vi "main.vi"() -> ()   [LabVIEW 2014]
uses:
  <vilib>/Instr/_visa.llb/VISA Configure Serial Port (Instr).vi
  <instrlib>/Keithley 24XX/Public/Data/Read (Single Point).vi
  <instrlib>/Keithley 24XX/Keithley 24XX.lvlib
panel:
  out "Seconds":sgl
  out "Chamber *C Data":string
  in  "Chamber *C Data":path=path "C:/Users/Administrator/Documents/humidity_sensing_setup/data/dumb/chamber_c_data.txt"
  out "Chamber *C Graph":sgl(graph)=5460.51
  out "Chamber *C":sgl
  out "Thermocouple Temperature Graph":sgl(graph)=5460.51
  out "Thermocouple Temperature":sgl
  out "Thermocouple *C Data":string
  in  "Thermocouple *C Data":path=path "C:/Users/Administrator/Documents/humidity_sensing_setup/data/dumb/thermocouple_c_data.txt"
  out "Pressure Data":string
  in  "Pressure Data":path=path "C:/Users/Administrator/Documents/humidity_sensing_setup/data/dumb/pressure_data.txt"
  out "Pressure Graph":sgl(graph)=5460.51
  out "Pressure":sgl
  in  "Start Button":bool
  in  "Operation Mode":bool
  out "Humidity":sgl
  out "Humidity Data":string
  in  "Humidity Data":path=path "C:/Users/Administrator/Documents/humidity_sensing_setup/data/dumb/humidity_data.txt"
  out "Humidity Data Graph":sgl(graph)=5460.51
  out "Resistance Data":string
  in  "Resistance Data":path=path "C:/Users/Administrator/Documents/humidity_sensing_setup/data/dumb/resistance_data.txt"
  out "Current Data":string
  in  "Current Data":path=path "C:/Users/Administrator/Documents/humidity_sensing_setup/data/dumb/current_data.txt"
  in  "Sampling rate (ms/pt)":i32=1000
  in  "Stop Voltage/Current":dbl=1.0
  in  "Start Voltage/Current":dbl=1.0
  in  "current multiplier":dbl=1000000.0
  in  "stop button":bool
  out "Current Data Graph":sgl(graph)=0.0001831192
  out "Resistance Data Graph":sgl(graph)=5460.51
  in  "loop num":dbl=10000000000.0
  in  "Step":dbl
  in  "Source Mode  (0: Voltage)":u16(ring) items=["Voltage", "Current"]
  in  "Compliance  Level (0.1)":dbl=1.0
  in  "Enable Resistance Auto R. (T:Enable)":bool
  in  "Enable Current Auto R. (T:Enable)":bool=TRUE
  in  "Enable Voltage Auto R. (T:Enable)":bool
  in  "Resistance M. R. (1.0)":dbl=1.0
  in  "Current M. Range (1.0)":dbl=1.0
  in  "Voltage M. Range (1.0)":dbl=1.0
  out "Resistance":sgl
  out "Current":sgl
  out "Voltage":sgl
  in  "Serial Configuration":T1={"Baud Rate"=9600, "Parity"=0, "Data Bits"=8, "Stop Bits"=10, "Flow Control"=0} {"Flow Control" items=["None", "XON/XOFF", "RTS/CTS", "XON/XOFF & RTS/CTS", "DTR/DSR", "XON/XOFF & DTR/DSR"]; "Stop Bits" items=["1.0"=10, "1.5"=15, "2.0"=20]; "Data Bits" items=["7"=7, "8"=8]; "Parity" items=["None", "Odd", "Even", "Mark", "Space"]; "Baud Rate" items=["300"=300, "600"=600, "1200"=1200, "2400"=2400, "4800"=4800, "9600"=9600, "19200"=19200]}
  in  "Keithley VISA resource name":refnum<visa-resource-name>="GPIB9::24::INSTR"
  out "Arduino Status":bool
  out "error out":errorcluster
  in  "error in":errorcluster
  in  "instr name":string="Arduino"
  in  "write":bool
  in  "buffer size":u32=256
  in  "timeout (ms)":u32=10000
  in  "flow control":u16
  in  "stop bits":u16=10
  in  "parity":u16(ring) items=["None", "Odd", "Even", "Mark", "Space"]
  in  "data bits":u16=8 min=5 max=8 step=1
  in  "baud rate":u32=9600
  in  "write string":string
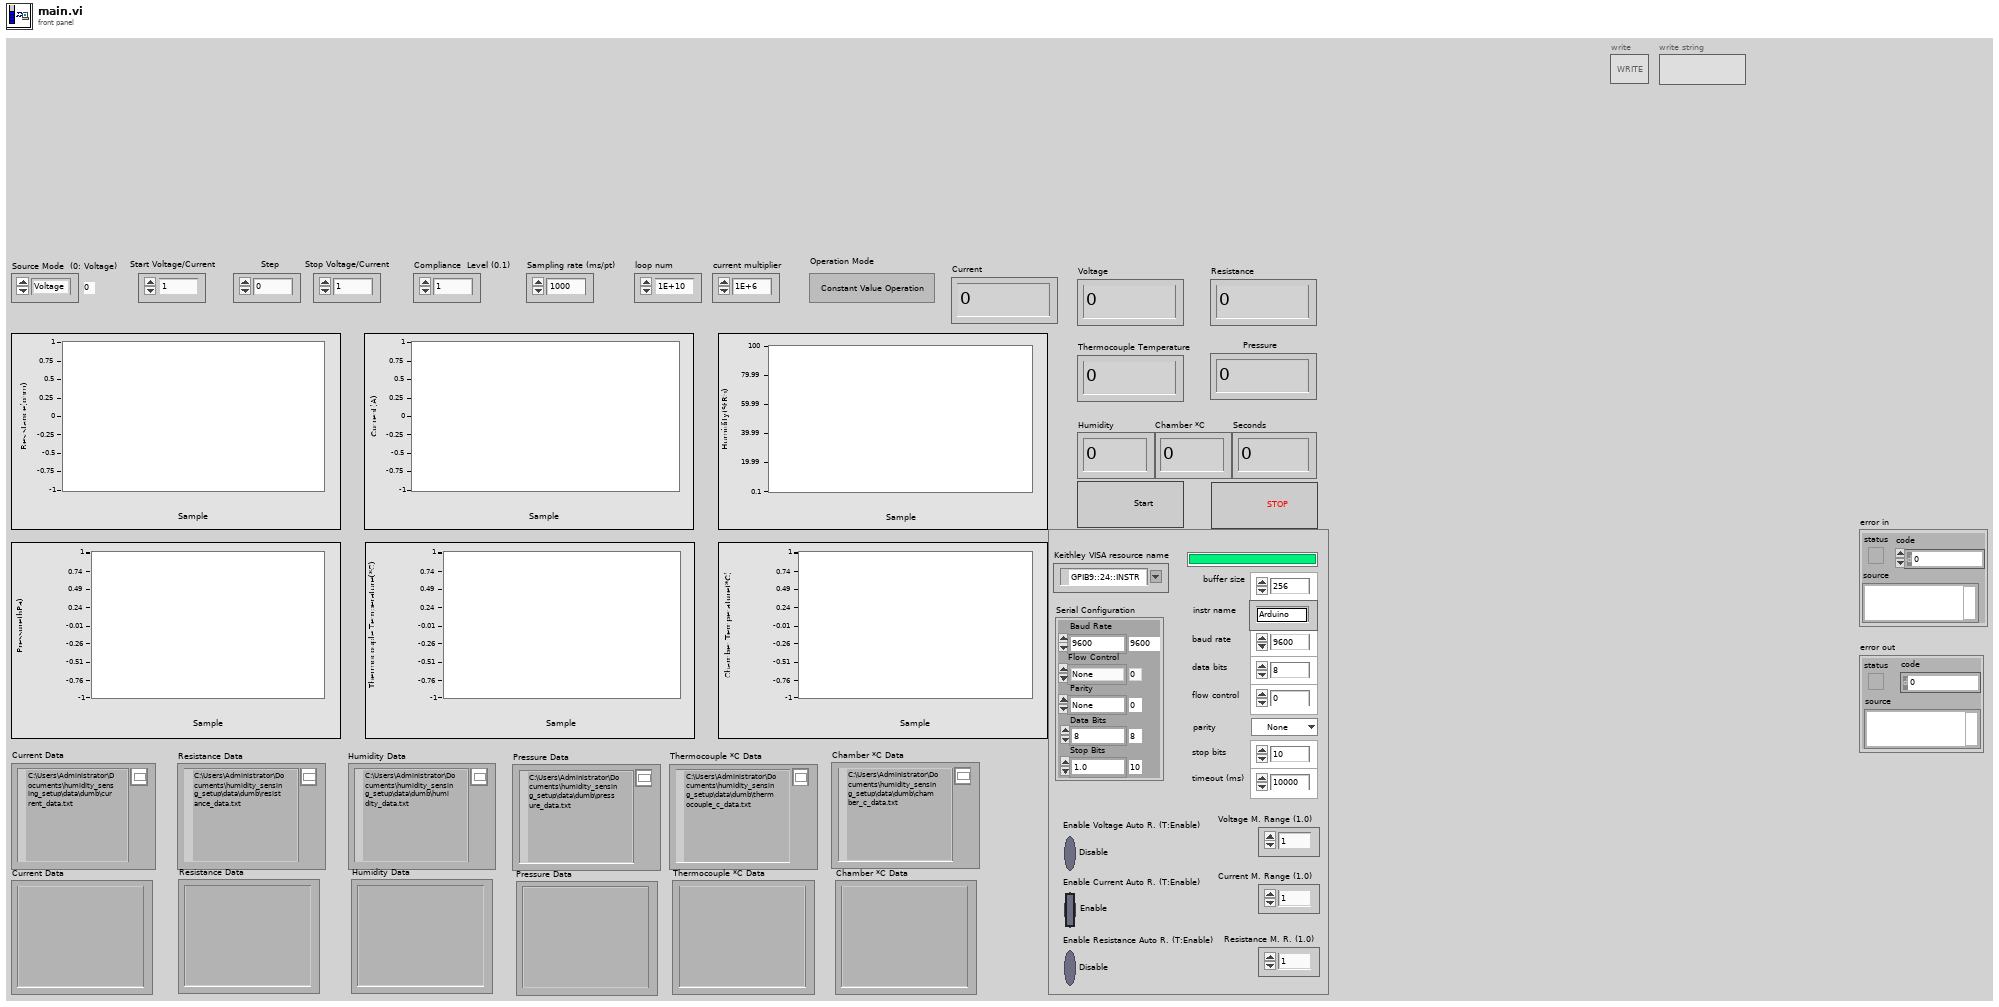
[diagram p1: front panel]
types:
  T1 = cluster{"Baud Rate":u32, "Parity":u16, "Data Bits":u16, "Stop Bits":u16, "Flow Control":u16}
  T2 = enum16{"open", "replace", "create", "open or create", "replace or create", "replace or create with confirmation"}
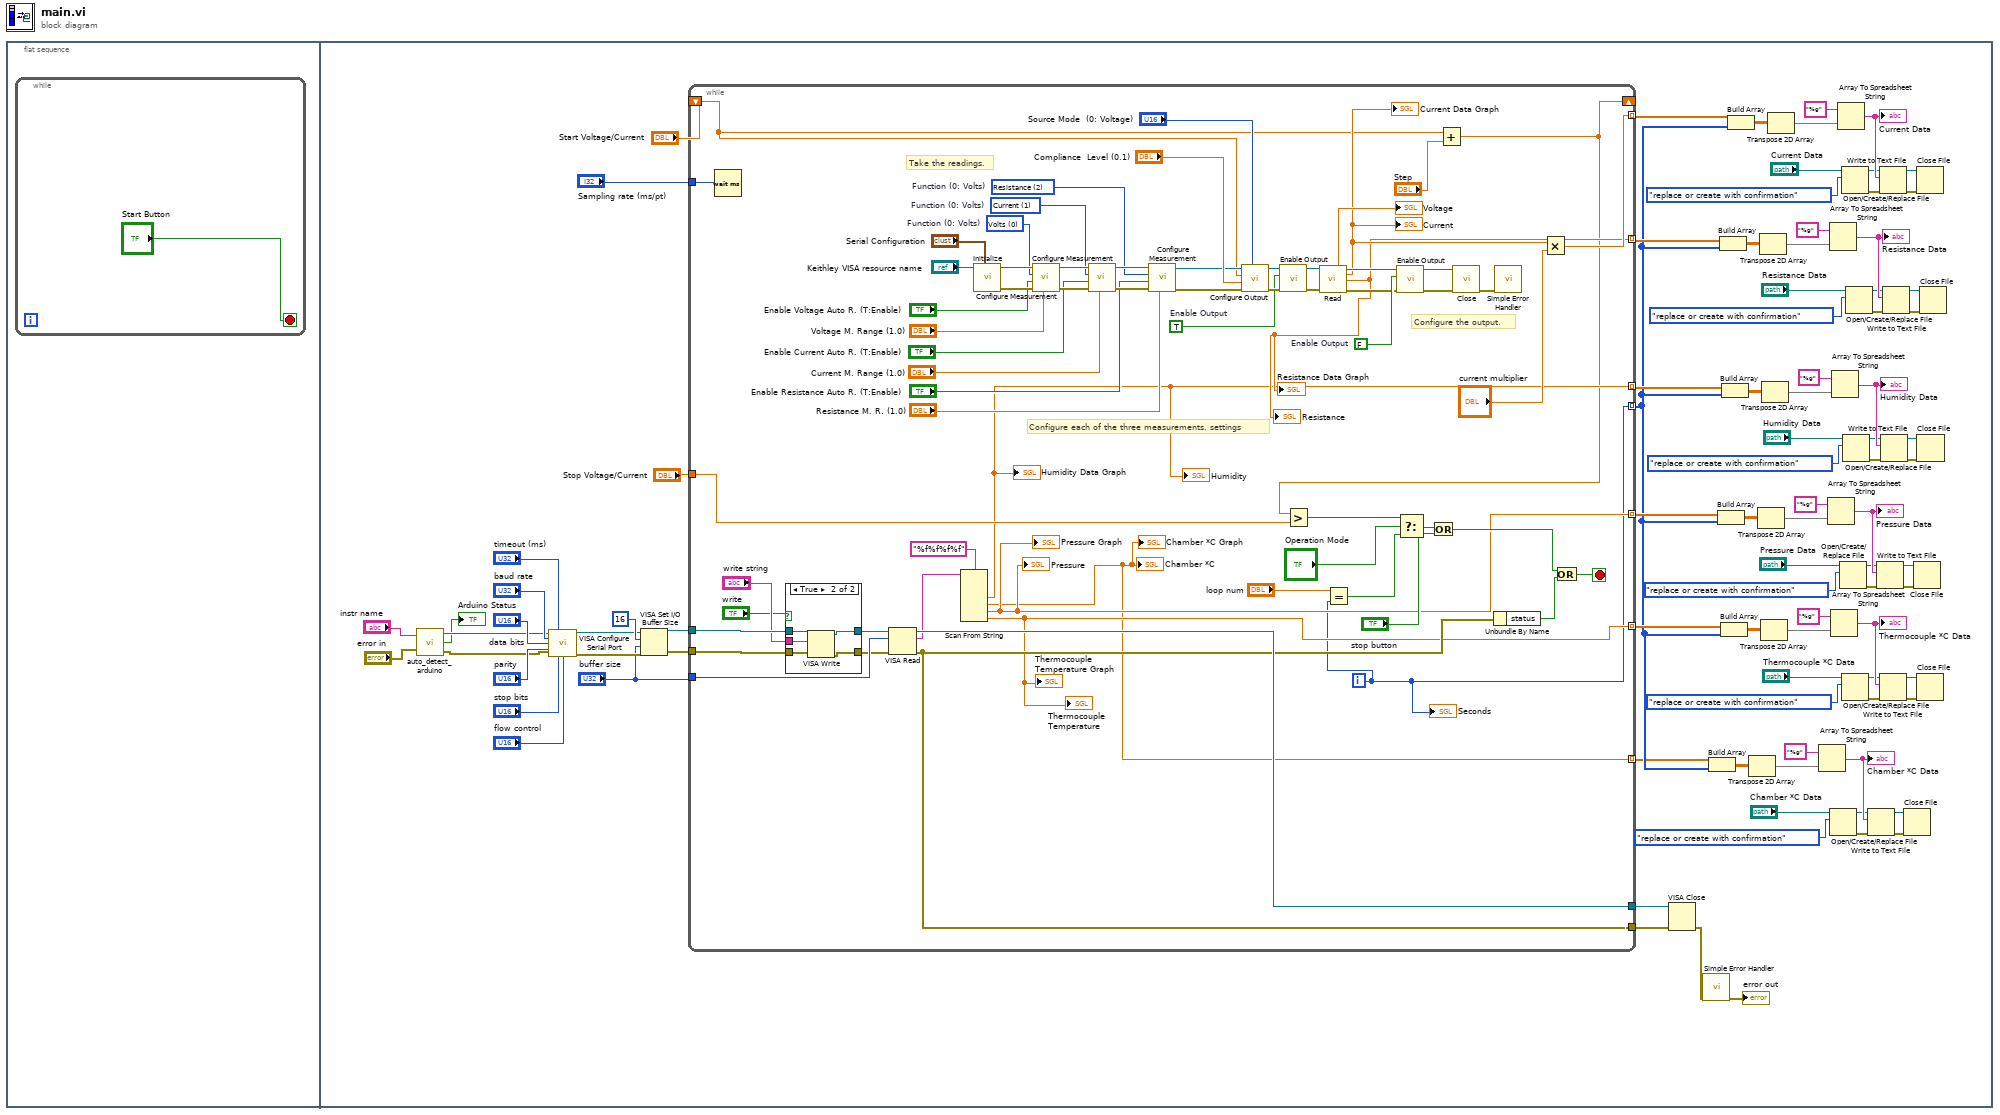
[diagram p0: block diagram]
diagram:
  n1 = flat-sequence {
    frame #0 {
      n2 = while {
        stop <- "Start Button" stop-if-true
      }
    }
    frame #1 {
      n3 = call "auto_detect_arduino.vi"("instr name"="instr name", "error in"="error in") -> ("VISA resource name"=w84:refnum<visa-resource-name>, "status"=→"Arduino Status":bool, "error out"=w83:errorcluster)
      n4 = call-poly "VISA Configure Serial Port"("VISA resource name"=w84, "timeout (10sec)"="timeout (ms)", "baud rate (9600)"="baud rate", "data bits (8)"="data bits", "parity (0:none)"="parity", "error in (no error)"=w83, "stop bits (10: 1 bit)"="stop bits", "flow control (0:none)"="flow control") -> ("VISA resource name out"=w80:refnum<visa-resource-name>, "error out"=w79:errorcluster)  [unwired: 6 in]
      n5 = VISA Set I/O Buffer Size(VISA resource name=w80, mask (16)=u16 16 ("I/O Receive\nBuffer mask"), size (4096)="buffer size", error in (no error)=w79) -> (VISA resource name out=w78:refnum<visa-resource-name>, error out=w77:errorcluster)
      n6 = while {
        tunnel: w78 -> [w156]
        tunnel: w77 -> [w155]
        tunnel: [w157] -> w92
        tunnel: [w100] -> w91
        tunnel: "buffer size" -> [w158]
        tunnel: [w102] -> w36 mode=indexing
        tunnel: "Sampling rate (ms/pt)" -> [w112]
        tunnel: "Stop Voltage/Current" -> [w111]
        tunnel: [w110] -> w49 mode=indexing
        tunnel: [w93] -> w3 mode=indexing
        tunnel: [w109] -> w48 mode=indexing
        shift-right: [w101] -> _
        shift-left: "Start Voltage/Current" -> [w108]
        tunnel: [w96] -> w25 mode=indexing
        tunnel: [w95] -> w14 mode=indexing
        tunnel: [w94] -> w2 mode=indexing
        i -> [w93]
        stop <- w159 stop-if-true
        w121 = TRUE  # Enable Output
        w131 = FALSE  # Enable Output
        w138 = u16 2 items=["Volts", "Current", "Resistance"]  # Function (0: Volts)
        w139 = u16 1 items=["Volts", "Current", "Resistance"]  # Function (0: Volts)
        w140 = u16 0 items=["Volts", "Current", "Resistance"]  # Function (0: Volts)
        # "Take the readings."
        # "Configure the output."
        # "Configure each of the three measurements. settings"
        n7 = Wait (ms)(milliseconds to wait=w112) -> ()  [unwired: 1 out]
        n8 = case shown="True" "write" {
          tunnel: w156 -> [w161 w166]
          tunnel: w155 -> [w160 w165]
          tunnel: [w161 w164] -> w154
          tunnel: [w160 w163] -> w153
          tunnel: "write string" -> [_ w162]
          frame False {
          }
          frame True {
            n9 = VISA Write(VISA resource name=w166, write buffer=w162, error in (no error)=w165) -> (VISA resource name out=w164:refnum<visa-resource-name>, error out=w163:errorcluster)  [unwired: 1 out]
          }
        }
        n10 = VISA Read(VISA resource name=w154, byte count=w158, error in (no error)=w153) -> (VISA resource name out=w157:refnum<visa-resource-name>, read buffer=w97:string, error out=w100:errorcluster)  [unwired: 1 out]
        n11 = Scan From String(format string="%f%f%f%f", input string=w97) -> (output 1=w102:sgl, output 2=w94:sgl, output 3=w96:sgl, output 4=w95:sgl)  [unwired: 6 in, 3 out]
        "Humidity Data Graph" <- w102
        "Humidity" <- w102
        "Pressure" <- w96
        "Pressure Graph" <- w96
        "Thermocouple Temperature" <- w95
        "Thermocouple Temperature Graph" <- w95
        "Chamber *C" <- w94
        "Chamber *C Graph" <- w94
        n12 = call <instrlib>:"Initialize.vi"("Serial Configuration"="Serial Configuration", "VISA resource name"="Keithley VISA resource name") -> ("error out"=w145:errorcluster, "VISA resource name out"=w146:refnum<visa-resource-name>)  [unwired: 8 in]
        n13 = call <instrlib>:"Configure Measurement.vi"("Manual Range (1.0)"="Voltage M. Range (1.0)", "error in (no error)"=w145, "Enable Auto Range (T:Enable)"="Enable Voltage Auto R. (T:Enable)", "Function (0: Volts)"=w140, "VISA resource name"=w146) -> ("error out"=w143:errorcluster, "VISA resource name out"=w144:refnum<visa-resource-name>)  [unwired: 5 in]
        n14 = call <instrlib>:"Configure Measurement.vi"("Manual Range (1.0)"="Current M. Range (1.0)", "error in (no error)"=w143, "Enable Auto Range (T:Enable)"="Enable Current Auto R. (T:Enable)", "Function (0: Volts)"=w139, "VISA resource name"=w144) -> ("error out"=w142:errorcluster, "VISA resource name out"=w141:refnum<visa-resource-name>)  [unwired: 5 in]
        n15 = call <instrlib>:"Configure Measurement.vi"("Manual Range (1.0)"="Resistance M. R. (1.0)", "error in (no error)"=w142, "Enable Auto Range (T:Enable)"="Enable Resistance Auto R. (T:Enable)", "Function (0: Volts)"=w138, "VISA resource name"=w141) -> ("error out"=w120:errorcluster, "VISA resource name out"=w119:refnum<visa-resource-name>)  [unwired: 5 in]
        n16 = call <instrlib>:"Configure Output.vi"("Source Mode  (0: Voltage)"="Source Mode  (0: Voltage)", "error in (no error)"=w120, "Compliance  Level (0.1)"="Compliance  Level (0.1)", "Output Level (0)"=w108, "VISA resource name"=w119) -> ("error out"=w122:errorcluster, "VISA resource name out"=w123:refnum<visa-resource-name>)  [unwired: 5 in]
        n17 = call <instrlib>:"Enable Output.vi"("error in (no error)"=w122, "Enable Output (T: Enable)"=w121, "VISA resource name"=w123) -> ("error out"=w125:errorcluster, "VISA resource name out"=w124:refnum<visa-resource-name>)  [unwired: 7 in]
        n18 = call-poly <instrlib>:"Read.vi"("VISA resource name"=w124, "error in (no error)"=w125) -> ("Voltage"=→"Voltage":sgl, "VISA resource name out"=w126:refnum<visa-resource-name>, "Current"=w114:sgl, "Resistance"=w109:sgl, "error out"=w127:errorcluster)  [unwired: 7 in, 2 out]
        "Current" <- w114
        "Resistance" <- w109
        "Resistance Data Graph" <- w109
        "Current Data Graph" <- w114
        n19 = Equal?(x="loop num", y=w93) -> (x = y?=w103:bool)
        n20 = call <instrlib>:"Enable Output.vi"("error in (no error)"=w127, "Enable Output (T: Enable)"=w131, "VISA resource name"=w126) -> ("error out"=w128:errorcluster, "VISA resource name out"=w129:refnum<visa-resource-name>)  [unwired: 7 in]
        n21 = Add(x=w108, y="Step") -> (x+y=w101:dbl)
        n22 = Greater?(x=w101, y=w111) -> (0:w106:bool)
        n23 = Select(t=w106, s="Operation Mode", f=w103) -> (s? t:f=w105:bool)
        n24 = Or(x=w105, y="stop button") -> (x .or. y?=w98:bool)
        n25 = call <instrlib>:"Close.vi"("error in (no error)"=w128, "VISA resource name"=w129) -> ("error out"=w149:errorcluster)  [unwired: 9 in]
        n26 = Unbundle By Name(w100) -> ("status"=w99:bool)
        n27 = call <vilib>:"Simple Error Handler.vi"("error in (no error)"=w149) -> ()  [unwired: 4 in, 5 out]
        n28 = Multiply(x=w114, y="current multiplier") -> (x*y=w110:dbl)
        n29 = Or(x=w98, y=w99) -> (x .or. y?=w159:bool)
        "Seconds" <- w93
      }
      n30 = VISA Close(VISA resource name=w92, error in (no error)=w91) -> (error out=w74:errorcluster)
      n31 = call <vilib>:"Simple Error Handler.vi"("error in (no error)"=w74) -> ("error out"=→"error out":errorcluster)  [unwired: 4 in, 4 out]
      n32 = Build Array(w2, w3) -> (w4:sgl[][])
      n33 = Build Array(w25, w3) -> (w26:sgl[][])
      n34 = Build Array(w48, w3) -> (w50:sgl[][])
      n35 = Build Array(w14, w3) -> (w15:sgl[][])
      n36 = Build Array(w36, w3) -> (w37:sgl[][])
      n37 = Build Array(w49, w3) -> (w66:dbl[][])
      n38 = Transpose 2D Array(2D array=w4) -> (transposed array=w12:sgl[][])
      n39 = Transpose 2D Array(2D array=w26) -> (transposed array=w34:sgl[][])
      n40 = Transpose 2D Array(2D array=w50) -> (transposed array=w58:sgl[][])
      n41 = Transpose 2D Array(2D array=w15) -> (transposed array=w23:sgl[][])
      n42 = Transpose 2D Array(2D array=w37) -> (transposed array=w45:sgl[][])
      n43 = Transpose 2D Array(2D array=w66) -> (transposed array=w68:dbl[][])
      n44 = Array To Spreadsheet String(array=w12, 3:"%g" ("format string")) -> (spreadsheet string=w13:string)  [unwired: 1 in]
      "Chamber *C Data" <- w13
      n45 = Array To Spreadsheet String(array=w34, 3:"%g" ("format string")) -> (spreadsheet string=w35:string)  [unwired: 1 in]
      "Pressure Data" <- w35
      n46 = Array To Spreadsheet String(array=w58, 3:"%g" ("format string")) -> (spreadsheet string=w59:string)  [unwired: 1 in]
      "Resistance Data" <- w59
      n47 = Open/Create/Replace File(file path (use dialog)="Chamber *C Data", operation (0:open)=T2."replace or create with confirmation") -> (refnum out=w10:refnum<file>, error out=w5:errorcluster)  [unwired: 4 in, 1 out]
      n48 = Array To Spreadsheet String(array=w23, 3:"%g" ("format string")) -> (spreadsheet string=w24:string)  [unwired: 1 in]
      "Thermocouple *C Data" <- w24
      n49 = Array To Spreadsheet String(array=w45, 3:"%g" ("format string")) -> (spreadsheet string=w46:string)  [unwired: 1 in]
      "Humidity Data" <- w46
      n50 = Array To Spreadsheet String(array=w68, 3:"%g" ("format string")) -> (spreadsheet string=w69:string)  [unwired: 1 in]
      "Current Data" <- w69
      n51 = Open/Create/Replace File(file path (use dialog)="Pressure Data", operation (0:open)=T2."replace or create with confirmation") -> (refnum out=w32:refnum<file>, error out=w27:errorcluster)  [unwired: 4 in, 1 out]
      n52 = Open/Create/Replace File(file path (use dialog)="Current Data", operation (0:open)=T2."replace or create with confirmation") -> (refnum out=w65:refnum<file>, error out=w60:errorcluster)  [unwired: 4 in, 1 out]
      n53 = Open/Create/Replace File(file path (use dialog)="Thermocouple *C Data", operation (0:open)=T2."replace or create with confirmation") -> (refnum out=w21:refnum<file>, error out=w16:errorcluster)  [unwired: 4 in, 1 out]
      n54 = Open/Create/Replace File(file path (use dialog)="Humidity Data", operation (0:open)=T2."replace or create with confirmation") -> (refnum out=w43:refnum<file>, error out=w38:errorcluster)  [unwired: 4 in, 1 out]
      n55 = Open/Create/Replace File(file path (use dialog)="Resistance Data", operation (0:open)=T2."replace or create with confirmation") -> (refnum out=w56:refnum<file>, error out=w51:errorcluster)  [unwired: 4 in, 1 out]
      n56 = Write to Text File(file (use dialog)=w10, text=w13, error in=w5) -> (refnum out=w7:refnum<file>, error out=w6:errorcluster)  [unwired: 2 out]
      n57 = Write to Text File(file (use dialog)=w32, text=w35, error in=w27) -> (refnum out=w29:refnum<file>, error out=w28:errorcluster)  [unwired: 2 out]
      n58 = Write to Text File(file (use dialog)=w65, text=w69, error in=w60) -> (refnum out=w62:refnum<file>, error out=w61:errorcluster)  [unwired: 2 out]
      n59 = Write to Text File(file (use dialog)=w21, text=w24, error in=w16) -> (refnum out=w18:refnum<file>, error out=w17:errorcluster)  [unwired: 2 out]
      n60 = Write to Text File(file (use dialog)=w43, text=w46, error in=w38) -> (refnum out=w40:refnum<file>, error out=w39:errorcluster)  [unwired: 2 out]
      n61 = Write to Text File(file (use dialog)=w56, text=w59, error in=w51) -> (refnum out=w53:refnum<file>, error out=w52:errorcluster)  [unwired: 2 out]
      n62 = Close File(refnum=w7, error in=w6) -> ()  [unwired: 2 out]
      n63 = Close File(refnum=w29, error in=w28) -> ()  [unwired: 2 out]
      n64 = Close File(refnum=w62, error in=w61) -> ()  [unwired: 2 out]
      n65 = Close File(refnum=w18, error in=w17) -> ()  [unwired: 2 out]
      n66 = Close File(refnum=w40, error in=w39) -> ()  [unwired: 2 out]
      n67 = Close File(refnum=w53, error in=w52) -> ()  [unwired: 2 out]
    }
  }
